vi "dfd_Render ZPK Equation.vi"(5 "fonts input":T3(array[cluster])=[{"Font Name:"="tahoma", "Size"=13, "Strikeout?"=FALSE, "Italic?"=FALSE, "Underline?"=FALSE, "Outline?"=TRUE, "Shadow?"=FALSE, "Bold?"=FALSE}, {"Font Name:"="tahoma", "Size"=13, "Strikeout?"=FALSE, "Italic?"=FALSE, "Underline?"=FALSE, "Outline?"=TRUE, "Shadow?"=FALSE, "Bold?"=FALSE}, {"Font Name:"="tahoma", "Size"=11, "Strikeout?"=FALSE, "Italic?"=FALSE, "Underline?"=FALSE, "Outline?"=TRUE, "Shadow?"=FALSE, "Bold?"=FALSE}], 6 "display format":T1 items=["Separated Roots", "Combined Roots"], 7 "format coeffiecients":string="%#_g", 8 "error in":errorcluster, 9 "origin":cluster{"left":i16, "top":i16}, 10 "ZPK coefficients":T2 {"gain" format="%.2f"; "poles" format="%.2f"; "zeroes" format="%.2f"}, 11 "picture in":picture) -> (0 "error out":errorcluster, 1 "size":cluster{"width":i16, "height":i16}, 3 "picture out":picture)   [LabVIEW 2017, in "NI_DigFilter_Process.lvlib"]
uses:
  <vilib>/addons/Digital Filter Design/NI_DigFilter_Process.lvlib
  <vilib>/addons/Digital Filter Design/Render.llb/dfd_ZPK Display Format.ctl
panel:
  in  "variable":string="z"
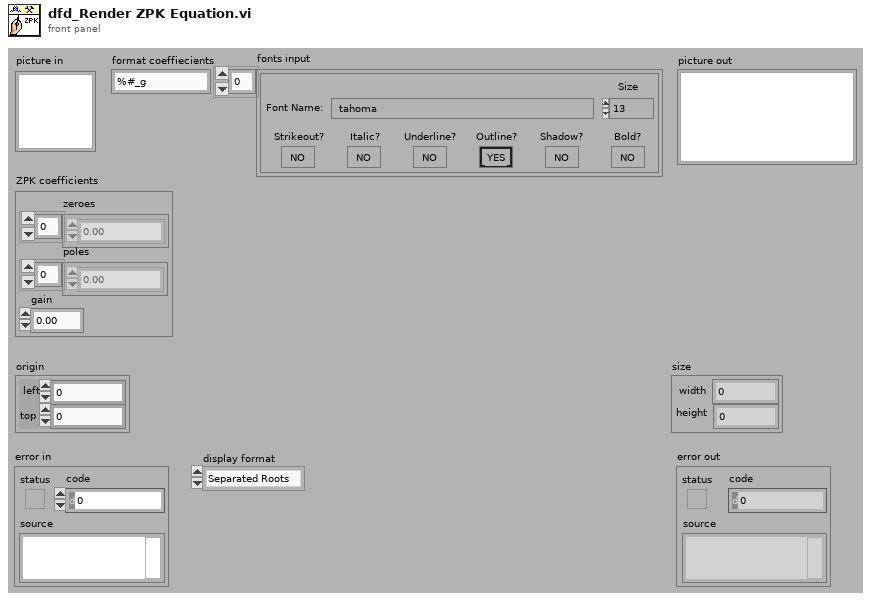
[diagram p1: front panel]
types:
  T1 = typedef "dfd_ZPK Display Format.ctl" = u16
  T2 = cluster{"zeroes":cdb[], "poles":cdb[], "gain":dbl}
  T3 = cluster{"Font Name:":string, "Size":i16, "Strikeout?":bool, "Italic?":bool, "Underline?":bool, "Outline?":bool, "Shadow?":bool, "Bold?":bool}[]
  T4 = cluster{"horizontal":enum16{"left", "center", "right"}, "vertical":enum16{"top", "center", "bottom"}}
  T5 = cluster{"left":i16, "top":i16, "right":i16, "bottom":i16}
  T6 = cluster{"Font Name:":string, "Size":i16, "Strikeout?":bool, "Italic?":bool, "Underline?":bool, "Outline?":bool, "Shadow?":bool, "Bold?":bool}
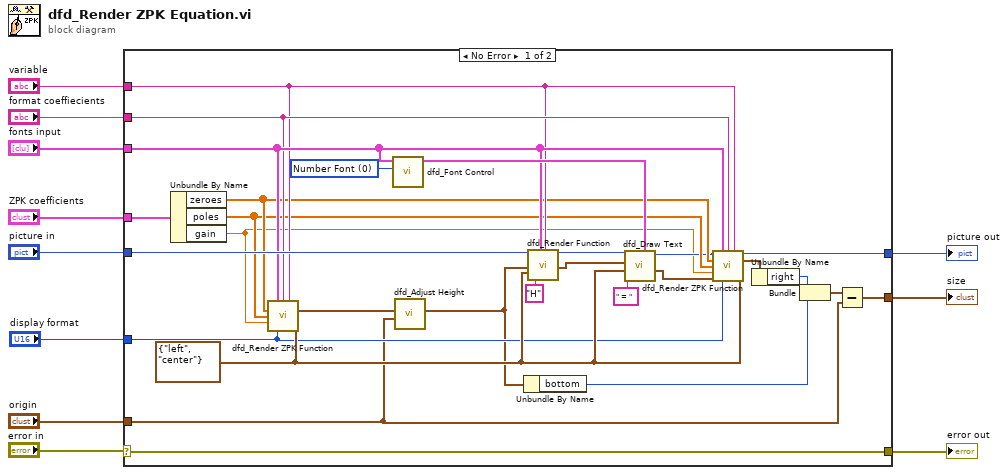
[diagram p0: block diagram]
diagram:
  n1 = case shown="No Error" "error in" {
    selector: "error in" -> [w32 w40]
    tunnel: "format coeffiecients" -> [w28 _]
    tunnel: "origin" -> [w14 _]
    tunnel: "picture in" -> [w36 _]
    tunnel: "variable" -> [w27 _]
    tunnel: "fonts input" -> [w29 _]
    tunnel: [w31 _] -> w2
    tunnel: "ZPK coefficients" -> [w33 _]
    tunnel: [w32 w40] -> w5
    tunnel: [w23 _] -> w4
    tunnel: "display format" -> [w16 _]
    frame No Error {
      w35 = u16 0 items=["Number Font", "Variable Font", "Script Font"] ("Tpye")
      w26 = T4 {"horizontal"=enum."left", "vertical"=enum."center"} ("alignment(left, top)")
      n2 = Unbundle By Name(w33) -> ("zeroes"=w22:cdb[], "poles"=w21:cdb[], "gain"=w19:dbl)
      n3 = call <vilib>:"dfd_Render ZPK Function.vi"("fonts input"=w29, "format coeffiecients"=w28, "variable"=w27, "numerator roots"=w22, "denominator roots"=w21, "gain"=w19, "alignment(left, top)"=w26, "display format"=w16) -> ("rect out"=w15:T5)  [unwired: 4 in, 3 out]
      n4 = call <vilib>:"dfd_Font Control.vi"("tpye"=w35, "fonts input"=w29) -> ("font output"=w34:T6)  [unwired: 9 out]
      n5 = call <vilib>:"dfd_Adjust Height.vi"("origin"=w14, "fraction rect"=w15) -> ("rect out"=w13:T5)  [unwired: 9 out]
      n6 = Unbundle By Name(w13) -> ("bottom"=w12:i16)
      n7 = call <vilib>:"dfd_Render Function.vi"("picture"=w36, "rect in"=w13, "alignment(left, top)"=w26, "function name"="H", "fonts input"=w29, "variable"=w27) -> ("new picture"=w39:picture, "rect out"=w37:T5)  [unwired: 4 in, 8 out]
      n8 = call <vilib>:"dfd_Draw Text.vi"("font input"=w34, "text"=" = ", "alignment(left, top)"=w26, "rect in"=w37, "picture in"=w39) -> ("rect out"=w17:T5, "picture out"=w20:picture)  [unwired: 3 in, 2 out]
      n9 = call <vilib>:"dfd_Render ZPK Function.vi"("picture in"=w20, "fonts input"=w29, "format coeffiecients"=w28, "variable"=w27, "numerator roots"=w22, "denominator roots"=w21, "gain"=w19, "alignment(left, top)"=w26, "rect in"=w17, "display format"=w16) -> ("picture out"=w31:picture, "rect out"=w30:T5)  [unwired: 2 in, 2 out]
      n10 = Unbundle By Name(w30) -> ("right"=w25:i16)
      n11 = Bundle("right"=w25, "bottom"=w12) -> (w24:cluster{"right":i16, "bottom":i16})  [unwired: 1 out]
      n12 = Subtract(x=w24, y=w14) -> (x-y=w23:cluster{i16, i16})
    }
    frame Error {
    }
  }
  "picture out" <- w2
  "error out" <- w5
  "size" <- w4
